vi "WSVCAP SHL FPGA LL Manage Initial States.vi"(0 "Transfer Cluster In":T1={"Transaction"=enum."I2C-Read Data", "Write Byte"=0, "Write Bits Remaining"=0, "Read Bits Remaining"=0, "Read Bytes Remaining"=0, "Wait Ticks Remaining"=0, "Slave Address"=0, "Bytes to Read"=2, "Bytes to Write"=0, "Sub Address"=2, "Socket Mask"=0, "Write CMD [1-4]"=0, "Write Bit Index [0-39]"=0, "CMD Delay (Ticks)"=0, "Commands per Cycle [1-4]"=0, "CMD Length [1-48]"=1, "Cycle Count"=2, "Cycle Mode"=TRUE, "CMD 1 Length (Bits)"=0, "CMD 2 Length (Bits)"=0, "CMD 3 Length (Bits)"=0, "CMD 4 Length (Bits)"=0, "CMD 1 Delay (Ticks)"=0, "CMD 2 Delay (Ticks)"=0, "CMD 3 Delay (Ticks)"=0, "CMD 4 Delay (Ticks)"=0, "CMD 1"=0, "CMD 2"=0, "CMD 3"=0, "CMD 4"=0, "Cycle CMD"=0, "Transaction Step"=enum."I2C Write - I:Send Slave Address", "Operation Step"=enum."I2C Send Slave Add - A: Send Start Sequence", "Procedure Step"=enum."I2C Start/Stop - 1: Set Clock Low", "Start Operation"=FALSE, "Start Procedure"=FALSE, "Procedure"=enum."I2C-Send Address Byte", "Wait Ticks"=2, "UUT Set (0/1)"=0} {"Cycle CMD" format="%.0x"; "CMD 4" format="%.0x"; "CMD 3" format="%.0x"; "CMD 2" format="%.0x"; "CMD 1" format="%.0x"; "Socket Mask" format="%012x"}) -> (4 "Transfer Cluster Out":T1={"Transaction"=enum."I2C-Read Data", "Write Byte"=0, "Write Bits Remaining"=0, "Read Bits Remaining"=0, "Read Bytes Remaining"=0, "Wait Ticks Remaining"=0, "Slave Address"=0, "Bytes to Read"=2, "Bytes to Write"=0, "Sub Address"=2, "Socket Mask"=0, "Write CMD [1-4]"=0, "Write Bit Index [0-39]"=0, "CMD Delay (Ticks)"=0, "Commands per Cycle [1-4]"=0, "CMD Length [1-48]"=1, "Cycle Count"=2, "Cycle Mode"=TRUE, "CMD 1 Length (Bits)"=0, "CMD 2 Length (Bits)"=0, "CMD 3 Length (Bits)"=0, "CMD 4 Length (Bits)"=0, "CMD 1 Delay (Ticks)"=0, "CMD 2 Delay (Ticks)"=0, "CMD 3 Delay (Ticks)"=0, "CMD 4 Delay (Ticks)"=0, "CMD 1"=0, "CMD 2"=0, "CMD 3"=0, "CMD 4"=0, "Cycle CMD"=0, "Transaction Step"=enum."I2C Write - I:Send Slave Address", "Operation Step"=enum."I2C Send Slave Add - A: Send Start Sequence", "Procedure Step"=enum."I2C Start/Stop - 1: Set Clock Low", "Start Operation"=FALSE, "Start Procedure"=FALSE, "Procedure"=enum."I2C-Send Address Byte", "Wait Ticks"=2, "UUT Set (0/1)"=0} {"Cycle CMD" format="%.0x"; "CMD 4" format="%.0x"; "CMD 3" format="%.0x"; "CMD 2" format="%.0x"; "CMD 1" format="%.0x"; "Socket Mask" format="%012x"})   [LabVIEW 2017]
uses:
  Type Defs/WSVCAP SHL Transaction Cluster.ctl
  Type Defs/WSVCAP SHL Transaction Enum.ctl
  Type Defs/WSVCAP SHL Transaction Step Enum.ctl
  Type Defs/WSVCAP SHL Operation Step Enum.ctl
  Type Defs/WSVCAP SHL Procedure Step Enum.ctl
  Type Defs/WSVCAP SHL Procedure Enum.ctl
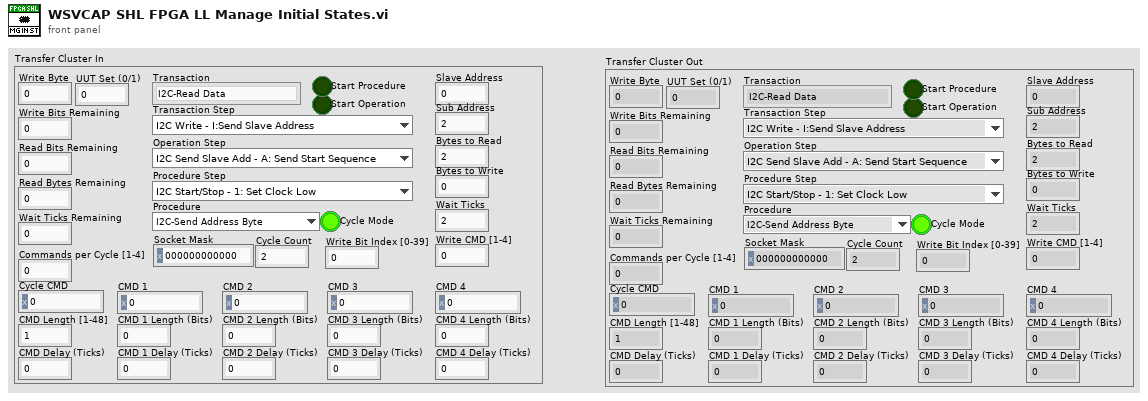
[diagram p1: front panel]
types:
  T1 = typedef "WSVCAP SHL Transaction Cluster.ctl" = cluster{"Transaction":T2, "Write Byte":u8, "Write Bits Remaining":u8, "Read Bits Remaining":u8, "Read Bytes Remaining":u8, "Wait Ticks Remaining":u32, "Slave Address":u8, "Bytes to Read":u8, "Bytes to Write":u8, "Sub Address":u8, "Socket Mask":u64, "Write CMD [1-4]":u8, "Write Bit Index [0-39]":u8, "CMD Delay (Ticks)":u32, "Commands per Cycle [1-4]":u8, "CMD Length [1-48]":u8, "Cycle Count":u64, "Cycle Mode":bool, "CMD 1 Length (Bits)":u8, "CMD 2 Length (Bits)":u8, "CMD 3 Length (Bits)":u8, "CMD 4 Length (Bits)":u8, "CMD 1 Delay (Ticks)":u32, "CMD 2 Delay (Ticks)":u32, "CMD 3 Delay (Ticks)":u32, "CMD 4 Delay (Ticks)":u32, "CMD 1":u64, "CMD 2":u64, "CMD 3":u64, "CMD 4":u64, "Cycle CMD":u64, "Transaction Step":T3, "Operation Step":T4, "Procedure Step":T5, "Start Operation":bool, "Start Procedure":bool, "Procedure":T6, "Wait Ticks":u32, "UUT Set (0/1)":u8}
  T2 = typedef "WSVCAP SHL Transaction Enum.ctl" = enum16{"I2C-Read Data", "I2C-Write Data", "RFFE-Ext Write", "RFFE-Ext Read"}
  T3 = typedef "WSVCAP SHL Transaction Step Enum.ctl" = enum16{"I2C Write - I:Send Slave Address", "I2C Write - II:Send Sub Address", "I2C Write - III:Send Data Bytes", "I2C Read - I:Send Slave Address (W)", "I2C Read - II:Send Sub Address", "I2C Read - III:Send Slave Address (R)", "I2C Read - IV:Read Data Bytes", "RFFE Ext Write - I.Write Data", "RFFE Ext Read - I:Read Data"}
  T4 = typedef "WSVCAP SHL Operation Step Enum.ctl" = enum16{"I2C Send Slave Add - A: Send Start Sequence", "I2C Send Slave Add - B: Load Address Byte", "I2C Send Slave Add - C: Send Address Byte", "I2C Send Slave Add - D: Read Slave ACK", "I2C Send Sub Add - A: Load Sub Address", "I2C Send Sub Add - B: Send Address Byte", "I2C Send Sub Add - C: Read Slave ACK", "I2C Send Data - A: Get Byte from FIFO", "I2C Send Data - B: Send Data Byte", "I2C Send Data - C: Read Slave ACK", "I2C Send Data - D: Send Stop Sequence", "I2C Read Data - A: Load Bytes to Read", "I2C Read Data - B: Receive Byte", "I2C Read Data - C: Write Master ACK", "I2C Read Data - D: Send Stop Sequence", "RFFE Read Data - A: Send SSC", "RFFE Read Data - B: Send CMD Frame", "RFFE Read Data - C: Receive Byte", "RFFE Write Data - A: Send SSC", "RFFE Write Data - B: Send Data", "RFFE Write Data - C: Wait CMD Delay", "RFFE Write Data - D: Clear Lines"}
  T5 = typedef "WSVCAP SHL Procedure Step Enum.ctl" = enum16{"I2C Start/Stop - 1: Set Clock Low", "I2C Start/Stop - 2: Wait", "I2C Start/Stop - 3: Set Data I", "I2C Start/Stop - 4: Wait", "I2C Start/Stop - 5: Set Clock High", "I2C Start/Stop - 6: Wait", "I2C Start/Stop - 7: Set Data II", "I2C Start/Stop - 8: Wait", "I2C Start/Stop - 9: Set Clock Low", "I2C Start/Stop - 10: Wait", "I2C Read ACK - 1: Set Clock High", "I2C Read ACK - 2: Wait", "I2C Read ACK - 3: Read ACK Bit", "I2C Read ACK - 4: Wait", "I2C Read ACK - 5: Set Clock Low", "I2C Read ACK - 6: Wait", "I2C Write ACK - 1: Write ACK Bit", "I2C Write ACK - 2: Wait", "I2C Write ACK - 3: Set Clock High", "I2C Write ACK - 4: Wait", "I2C Write ACK - 5: Set Clock Low", "I2C Write ACK - 6: Wait", "I2C Write ACK - 7: Set Data Low", "I2C Send Add - 1: Reset Bits Remaining", "I2C Send Add - 2: Set Data Bit", "I2C Send Add - 3: Wait", "I2C Send Add - 4: Set Clock High", "I2C Send Add - 5: Wait", "I2C Send Add - 6: Set Clock Low", "I2C Send Add - 7: Wait", "I2C Send Add - 8: Check Bits Remaining", "I2C Send Data - 1: Reset Bits Remaining", "I2C Send Data - 2: Load Write Bit from FIFO", "I2C Send Data - 3: Set Data Bit", "I2C Send Data - 4: Wait", "I2C Send Data - 5: Set Clock High", "I2C Send Data - 6: Wait", "I2C Send Data - 7: Set Clock Low", "I2C Send Data - 8: Wait", "I2C Send Data - 9: Check Bits Remaining", "I2C Receive Data - 1: Reset Bits Remaining", "I2C Receive Data - 2: Wait", "I2C Receive Data - 3: Set Clock High", "I2C Receive Data - 4: Wait", "I2C Receive Data - 5: Read Data Bit", "I2C Receive Data - 6: Wait", "I2C Receive Data - 7: Set Clock Low", "I2C Receive Data - 8: Wait", "I2C Receive Data - 9: Check Bits Remaining", "RFFE Send SSC - 1:Set Low", "RFFE Send SSC - 2:Wait", "RFFE Send SSC - 3:Set SDA High", "RFFE Send SSC - 4:Wait", "RFFE Send SSC - 5:Set SDA Low", "RFFE Send SSC - 6:Wait", "RFFE Send Data - 1:Set SCL High", "RFFE Send Data - 2:Wait", "RFFE Send Data - 3:Set SCL Low", "RFFE Send Data - 4:Wait", "RFFE Send Data - 5:Set SCL High (P)", "RFFE Send Data - 6:Wait", "RFFE Send Data - 7:Set SCL Low (P)", "RFFE Send Data - 8:Wait", "RFFE Send Data - 9:Set SCL High (BP)", "RFFE Send Data - 10:Wait", "RFFE Send Data - 11:Set SCL Low (BP)", "RFFE Send Data - 12:Wait", "RFFE Receive Data - 1:Set SCL High", "RFFE Receive Data - 2:Wait", "RFFE Receive Data - 3:Set SCL Low", "RFFE Receive Data - 4:Wait", "RFFE Receive Data - 5:Set SCL High (BP)", "RFFE Receive Data - 6:Wait", "RFFE Receive Data - 7:Set SCL Low (BP)", "RFFE Receive Data - 8:Wait", "RFFE Wait CMD Delay - 1:Wait", "RFFE Clear Lines - 1:Clear"}
  T6 = typedef "WSVCAP SHL Procedure Enum.ctl" = enum16{"None", "I2C-Send Start/Stop Sequence", "I2C-Send Address Byte", "I2C-Send Data Byte", "I2C-Read ACK", "I2C-Receive Byte", "I2C-Write ACK", "RFFE-Clear Lines", "RFFE-Send SSC", "RFFE-Send Data", "RFFE-Receive Data", "RFFE-Wait CMD Delay"}
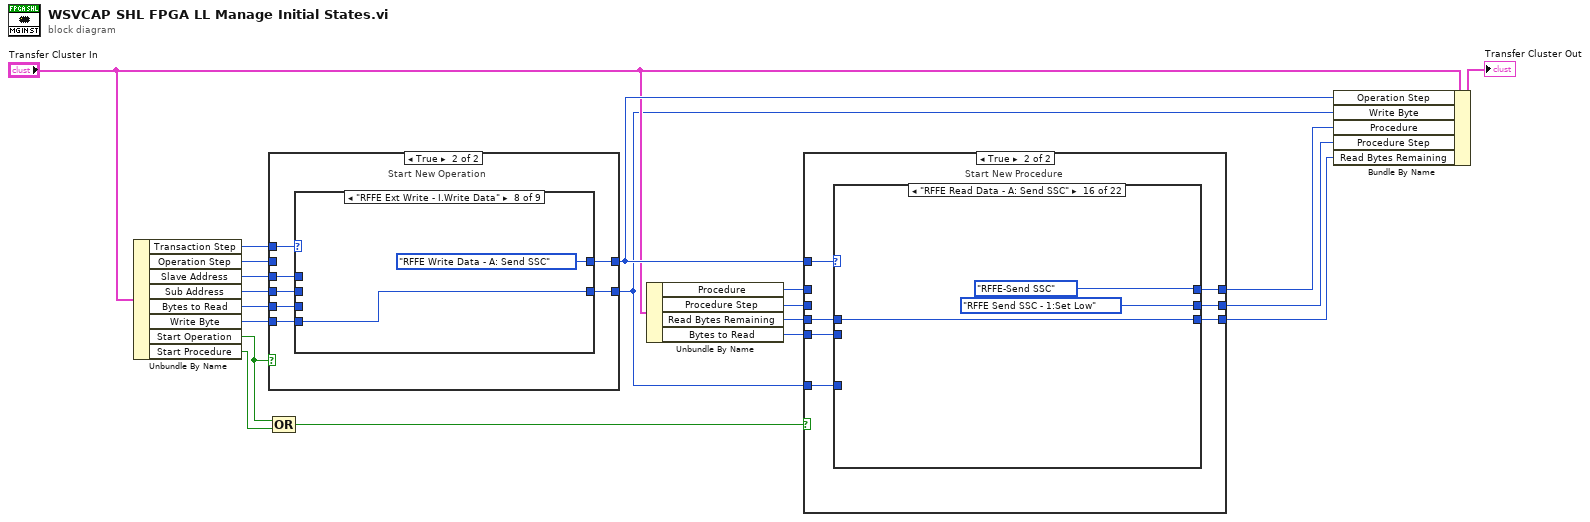
[diagram p0: block diagram]
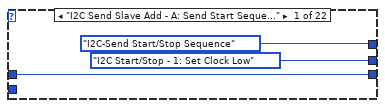
[diagram p3: hidden frame]
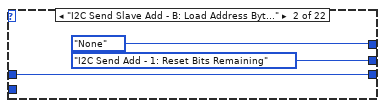
[diagram p4: hidden frame]
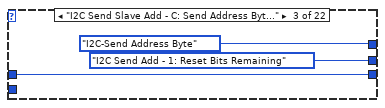
[diagram p5: hidden frame]
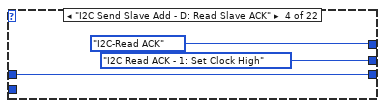
[diagram p6: hidden frame]
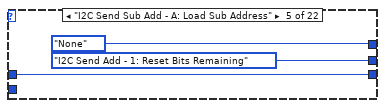
[diagram p7: hidden frame]
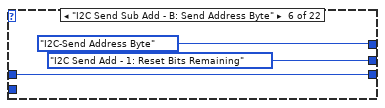
[diagram p8: hidden frame]
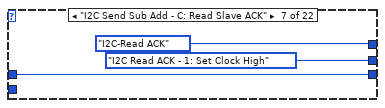
[diagram p9: hidden frame]
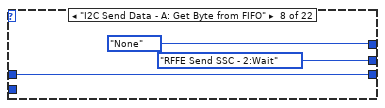
[diagram p10: hidden frame]
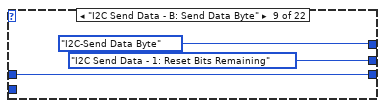
[diagram p11: hidden frame]
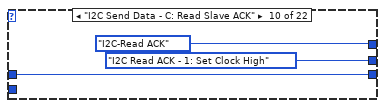
[diagram p12: hidden frame]
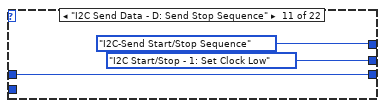
[diagram p13: hidden frame]
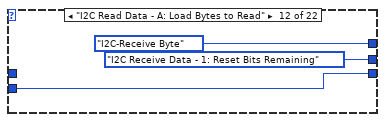
[diagram p14: hidden frame]
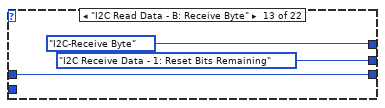
[diagram p15: hidden frame]
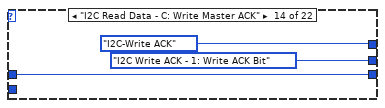
[diagram p16: hidden frame]
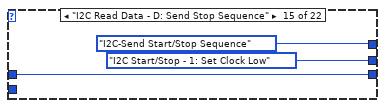
[diagram p17: hidden frame]
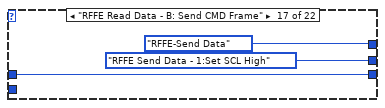
[diagram p18: hidden frame]
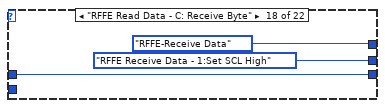
[diagram p19: hidden frame]
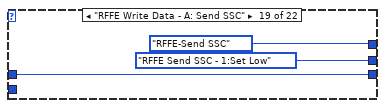
[diagram p20: hidden frame]
diagram:
  n1 = Unbundle By Name("Transfer Cluster In") -> ("Transaction Step"=w20:T3, "Operation Step"=w19:T4, "Slave Address"=w18:u8, "Sub Address"=w17:u8, "Bytes to Read"=w16:u8, "Write Byte"=w14:u8, "Start Operation"=w6:bool, "Start Procedure"=w5:bool)
  n2 = case shown="True" w6 {
    tunnel: w20 -> [_ w29]
    tunnel: [w22 w28] -> w13
    tunnel: w19 -> [w22 _]
    tunnel: w18 -> [_ w27]
    tunnel: w17 -> [_ w26]
    tunnel: w16 -> [_ w25]
    tunnel: [w21 w24] -> w1
    tunnel: w14 -> [w21 w23]
    frame False {
      # "Continue Current Operation"
    }
    frame True {
      # "Start New Operation"
      n3 = case shown="\"RFFE Ext Write - I.Write Data\"" w29 {
        tunnel: [WSVCAP_SHL_Operation_Step_Enum."I2C Send Slave Add - A: Send Start Sequence" ("Operation Step Out") WSVCAP_SHL_Operation_Step_Enum."I2C Send Sub Add - A: Load Sub Address" ("Operation Step Out") WSVCAP_SHL_Operation_Step_Enum."I2C Send Data - A: Get Byte from FIFO" ("Operation Step Out") WSVCAP_SHL_Operation_Step_Enum."I2C Send Slave Add - A: Send Start Sequence" ("Operation Step Out") WSVCAP_SHL_Operation_Step_Enum."I2C Send Sub Add - A: Load Sub Address" ("Operation Step Out") WSVCAP_SHL_Operation_Step_Enum."I2C Send Slave Add - A: Send Start Sequence" ("Operation Step Out") WSVCAP_SHL_Operation_Step_Enum."I2C Read Data - A: Load Bytes to Read" ("Operation Step Out") WSVCAP_SHL_Operation_Step_Enum."RFFE Write Data - A: Send SSC" ("Operation Step Out") WSVCAP_SHL_Operation_Step_Enum."RFFE Read Data - A: Send SSC" ("Operation Step Out")] -> w28
        tunnel: w27 -> [w30 _ _ w36 _ w41 _ _ _]
        tunnel: w26 -> [_ w32 _ _ w38 _ _ _ _]
        tunnel: w25 -> [_ _ _ _ _ _ _ _ _]
        tunnel: [w30 w32 w34 w36 w38 w40 w44 w46 w48] -> w24
        tunnel: w23 -> [_ _ w34 _ _ _ w44 w46 w48]
        frame "I2C Write - I:Send Slave Address" {
        }
        frame "I2C Write - II:Send Sub Address" {
        }
        frame "I2C Write - III:Send Data Bytes" {
        }
        frame "I2C Read - I:Send Slave Address (W)" {
        }
        frame "I2C Read - II:Send Sub Address" {
        }
        frame "I2C Read - III:Send Slave Address (R)" {
          n4 = Compound Arithmetic op=OR(w41, u8 1 ("value")) -> (w40:u8)
        }
        frame "I2C Read - IV:Read Data Bytes" {
        }
        frame "RFFE Ext Write - I.Write Data" {
        }
        frame "RFFE Ext Read - I:Read Data" {
        }
      }
    }
  }
  n5 = Compound Arithmetic op=OR(w6, w5) -> (w15:bool)
  n6 = Unbundle By Name("Transfer Cluster In") -> ("Procedure"=w3:T6, "Procedure Step"=w12:T5, "Read Bytes Remaining"=w9:u8, "Bytes to Read"=w8:u8)
  n7 = case shown="True" w15 {
    tunnel: w13 -> [_ w59]
    tunnel: [w52 w58] -> w10
    tunnel: w12 -> [w52 _]
    tunnel: w9 -> [w51 w57]
    tunnel: w8 -> [_ w56]
    tunnel: [w51 w55] -> w7
    tunnel: [w50 w54] -> w2
    tunnel: w3 -> [w50 _]
    tunnel: w1 -> [_ w53]
    frame False {
      # "Continue Current Procedure"
    }
    frame True {
      # "Start New Procedure"
      n8 = case shown="\"RFFE Read Data - A: Send SSC\"" w59 {
        tunnel: [WSVCAP_SHL_Procedure_Step_Enum."I2C Start/Stop - 1: Set Clock Low" ("Procedure Step Out") WSVCAP_SHL_Procedure_Step_Enum."I2C Send Add - 1: Reset Bits Remaining" ("Procedure Step Out") WSVCAP_SHL_Procedure_Step_Enum."I2C Send Add - 1: Reset Bits Remaining" ("Procedure Step Out") WSVCAP_SHL_Procedure_Step_Enum."I2C Read ACK - 1: Set Clock High" ("Procedure Step Out") WSVCAP_SHL_Procedure_Step_Enum."I2C Send Add - 1: Reset Bits Remaining" ("Procedure Step Out") WSVCAP_SHL_Procedure_Step_Enum."I2C Send Add - 1: Reset Bits Remaining" ("Procedure Step Out") WSVCAP_SHL_Procedure_Step_Enum."I2C Read ACK - 1: Set Clock High" ("Procedure Step Out") WSVCAP_SHL_Procedure_Step_Enum."RFFE Send SSC - 2:Wait" ("Procedure Step Out") WSVCAP_SHL_Procedure_Step_Enum."I2C Send Data - 1: Reset Bits Remaining" ("Procedure Step Out") WSVCAP_SHL_Procedure_Step_Enum."I2C Read ACK - 1: Set Clock High" ("Procedure Step Out") WSVCAP_SHL_Procedure_Step_Enum."I2C Start/Stop - 1: Set Clock Low" ("Procedure Step Out") WSVCAP_SHL_Procedure_Step_Enum."I2C Receive Data - 1: Reset Bits Remaining" ("Procedure Step Out") WSVCAP_SHL_Procedure_Step_Enum."I2C Receive Data - 1: Reset Bits Remaining" ("Procedure Step Out") WSVCAP_SHL_Procedure_Step_Enum."I2C Write ACK - 1: Write ACK Bit" ("Procedure Step Out") WSVCAP_SHL_Procedure_Step_Enum."I2C Start/Stop - 1: Set Clock Low" ("Procedure Step Out") WSVCAP_SHL_Procedure_Step_Enum."RFFE Send SSC - 1:Set Low" ("Procedure Step Out") WSVCAP_SHL_Procedure_Step_Enum."RFFE Send Data - 1:Set SCL High" ("Procedure Step Out") WSVCAP_SHL_Procedure_Step_Enum."RFFE Receive Data - 1:Set SCL High" ("Procedure Step Out") WSVCAP_SHL_Procedure_Step_Enum."RFFE Send SSC - 1:Set Low" ("Procedure Step Out") WSVCAP_SHL_Procedure_Step_Enum."RFFE Send Data - 1:Set SCL High" ("Procedure Step Out") WSVCAP_SHL_Procedure_Step_Enum."RFFE Wait CMD Delay - 1:Wait" ("Procedure Step Out") WSVCAP_SHL_Procedure_Step_Enum."RFFE Clear Lines - 1:Clear" ("Procedure Step Out")] -> w58
        tunnel: [w61 w64 w67 w70 w73 w76 w79 w82 w85 w88 w91 w94 w97 w100 w103 w106 w109 w112 w115 w118 w121 w124] -> w55
        tunnel: w57 -> [w61 w64 w67 w70 w73 w76 w79 w82 w85 w88 w91 _ w97 w100 w103 w106 w109 w112 w115 w118 w121 w124]
        tunnel: w56 -> [_ _ _ _ _ _ _ _ _ _ _ w94 _ _ _ _ _ _ _ _ _ _]
        tunnel: [WSVCAP_SHL_Procedure_Enum."I2C-Send Start/Stop Sequence" ("Procedure") WSVCAP_SHL_Procedure_Enum."None" ("Procedure") WSVCAP_SHL_Procedure_Enum."I2C-Send Address Byte" ("Procedure") WSVCAP_SHL_Procedure_Enum."I2C-Read ACK" ("Procedure") WSVCAP_SHL_Procedure_Enum."None" ("Procedure") WSVCAP_SHL_Procedure_Enum."I2C-Send Address Byte" ("Procedure") WSVCAP_SHL_Procedure_Enum."I2C-Read ACK" ("Procedure") WSVCAP_SHL_Procedure_Enum."None" ("Procedure") WSVCAP_SHL_Procedure_Enum."I2C-Send Data Byte" ("Procedure") WSVCAP_SHL_Procedure_Enum."I2C-Read ACK" ("Procedure") WSVCAP_SHL_Procedure_Enum."I2C-Send Start/Stop Sequence" ("Procedure") WSVCAP_SHL_Procedure_Enum."I2C-Receive Byte" ("Procedure") WSVCAP_SHL_Procedure_Enum."I2C-Receive Byte" ("Procedure") WSVCAP_SHL_Procedure_Enum."I2C-Write ACK" ("Procedure") WSVCAP_SHL_Procedure_Enum."I2C-Send Start/Stop Sequence" ("Procedure") WSVCAP_SHL_Procedure_Enum."RFFE-Send SSC" ("Procedure") WSVCAP_SHL_Procedure_Enum."RFFE-Send Data" ("Procedure") WSVCAP_SHL_Procedure_Enum."RFFE-Receive Data" ("Procedure") WSVCAP_SHL_Procedure_Enum."RFFE-Send SSC" ("Procedure") WSVCAP_SHL_Procedure_Enum."RFFE-Send Data" ("Procedure") WSVCAP_SHL_Procedure_Enum."RFFE-Wait CMD Delay" ("Procedure") WSVCAP_SHL_Procedure_Enum."RFFE-Clear Lines" ("Procedure")] -> w54
        tunnel: w53 -> [_ _ _ _ _ _ _ _ _ _ _ _ _ _ _ _ _ _ _ _ _ _]
        frame "I2C Send Slave Add - A: Send Start Sequence" {
        }
        frame "I2C Send Slave Add - B: Load Address Byte" {
        }
        frame "I2C Send Slave Add - C: Send Address Byte" {
        }
        frame "I2C Send Slave Add - D: Read Slave ACK" {
        }
        frame "I2C Send Sub Add - A: Load Sub Address" {
        }
        frame "I2C Send Sub Add - B: Send Address Byte" {
        }
        frame "I2C Send Sub Add - C: Read Slave ACK" {
        }
        frame "I2C Send Data - A: Get Byte from FIFO" {
        }
        frame "I2C Send Data - B: Send Data Byte" {
        }
        frame "I2C Send Data - C: Read Slave ACK" {
        }
        frame "I2C Send Data - D: Send Stop Sequence" {
        }
        frame "I2C Read Data - A: Load Bytes to Read" {
        }
        frame "I2C Read Data - B: Receive Byte" {
        }
        frame "I2C Read Data - C: Write Master ACK" {
        }
        frame "I2C Read Data - D: Send Stop Sequence" {
        }
        frame "RFFE Read Data - A: Send SSC" {
        }
        frame "RFFE Read Data - B: Send CMD Frame" {
        }
        frame "RFFE Read Data - C: Receive Byte" {
        }
        frame "RFFE Write Data - A: Send SSC" {
        }
        frame "RFFE Write Data - B: Send Data" {
        }
        frame "RFFE Write Data - C: Wait CMD Delay" {
        }
        frame "RFFE Write Data - D: Clear Lines" {
        }
      }
    }
  }
  n9 = Bundle By Name(cluster="Transfer Cluster In", "Operation Step"=w13, "Write Byte"=w1, "Procedure"=w2, "Procedure Step"=w10, "Read Bytes Remaining"=w7) -> (→"Transfer Cluster Out":T1)
